vi "Lockin_AIWFM_time.vi"(8 "error in (no error)":errorcluster, 11 "Transport":refnum<class "Transport.lvclass">) -> (0 "error out":errorcluster, 3 "Transport out":refnum<class "Transport.lvclass">)   [LabVIEW 2016, in "Transport.lvclass"]
uses:
  Transport.lvclass
  Control Experiment/Typedefs/Instruments--cluster.ctl
  <userlib>/LevyLab/Krohn Hite 7008/Instrument.KH7008.lvclass
  <userlib>/LevyLab/Lockin-Multichannel/Instrument.Lockin/Instrument.Lockin.lvclass
  <userlib>/LevyLab/Levylab Instruments/Instrument Types/Cryostat/Instrument.Cryostat.lvclass
  <userlib>/LevyLab/Levylab Instruments/Instrument Types/CBridge/Instrument.CBridge.lvclass
  <userlib>/LevyLab/Levylab Instruments/Instrument Types/Optical Delay Line/Instrument.OpticalDelayLine.lvclass
  <userlib>/LevyLab/Levylab Instruments/Instrument Types/Strain/Instrument.Strain.lvclass
  <userlib>/LevyLab/Levylab Instruments/Instrument Types/VNA/Instrument.VNA.lvclass
  <userlib>/LevyLab/Levylab Instruments/Instrument Types/VSource/Instrument.VSource.lvclass
  Transport.lvclass/Transport.ctl
  Control Experiment/Control Experiment.lvclass/Control Experiment.ctl
  <userlib>/LevyLab/XY Utilities/subVIs/Waveform to XY (single).vi
  <userlib>/LevyLab/XY Utilities/subVIs/Get X and Y (single).vi
  <vilib>/Waveform/WDTOps.llb/WDT Append Waveforms DBL.vi
  Control Experiment/Control Experiment.lvclass
  <userlib>/LevyLab/XY Utilities/xy_utilities.lvlib
panel:
  in  "Stop":bool
  in  "Tab Control":enum32{"Control", "Waveform", "Other"}(tab)
  in  "wait (ms)":u32=1000
  in  "Experiment Description":string="cool down\n\n"
  in  "Experiment Folder":string="cooldown"
  out "AI":cluster{dbl[], dbl[]}[](graph)
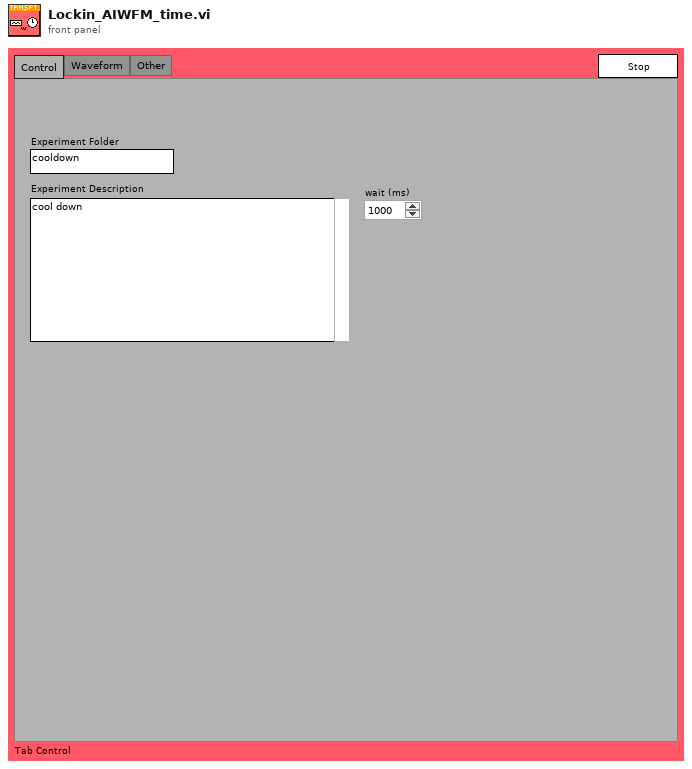
[diagram p1: front panel]
types:
  T1 = enum32{"Invalid", "Standard", "Closed", "Hidden", "Minimized", "Maximized"}
  T2 = enum32{"invalid app kind", "Development System", "Run Time System", "Student Edition", "Embedded LabVIEW", "Evaluation", "Custom"}
  T3 = typedef "Control Experiment.lvclass/Instruments--cluster.ctl" = cluster{"KH7008":refnum<class "Instrument.KH7008.lvclass">[], "Lockin":refnum<class "Instrument.Lockin.lvclass">, "Temperature":refnum<class "Instrument.Cryostat.lvclass">, "Magnet":refnum<class "Instrument.Cryostat.lvclass">, "Rotator":refnum<class "Instrument.Cryostat.lvclass">, "Level":refnum<class "Instrument.Cryostat.lvclass">, "Capacitance Bridge":refnum<class "Instrument.CBridge.lvclass">, "Optical Delay Line":refnum<class "Instrument.OpticalDelayLine.lvclass">, "Strain Cell":refnum<class "Instrument.Strain.lvclass">, "VNA":refnum<class "Instrument.VNA.lvclass">, "Voltage Source":refnum<class "Instrument.VSource.lvclass">}
  T4 = cluster{"Core":cluster{"Current VI Reference":refnum<vi>, "Close Panel on Exit?":bool}, "Transport":refnum<class "Transport.lvclass">, "SweepControl":refnum<class "SweepControl.lvclass">, "Control Experiment":refnum<class "Control Experiment.lvclass">, "Notifier":refnum<notifier>, "Instruments":T3, "path":path, "time":dbl, "temperature":dbl, "magnet field":dbl, "AI XY (new)":cluster{dbl[], dbl[]}[], "AI XY (all)":cluster{dbl[], dbl[]}[], "AI Waveform (s)":waveform(dbl)[], "t0":timestamp}
  T5 = cluster{"Current VI Reference":refnum<vi>, "Close Panel on Exit?":bool}
  T6 = enum32{"Bad", "Idle", "Run top level", "Running"}
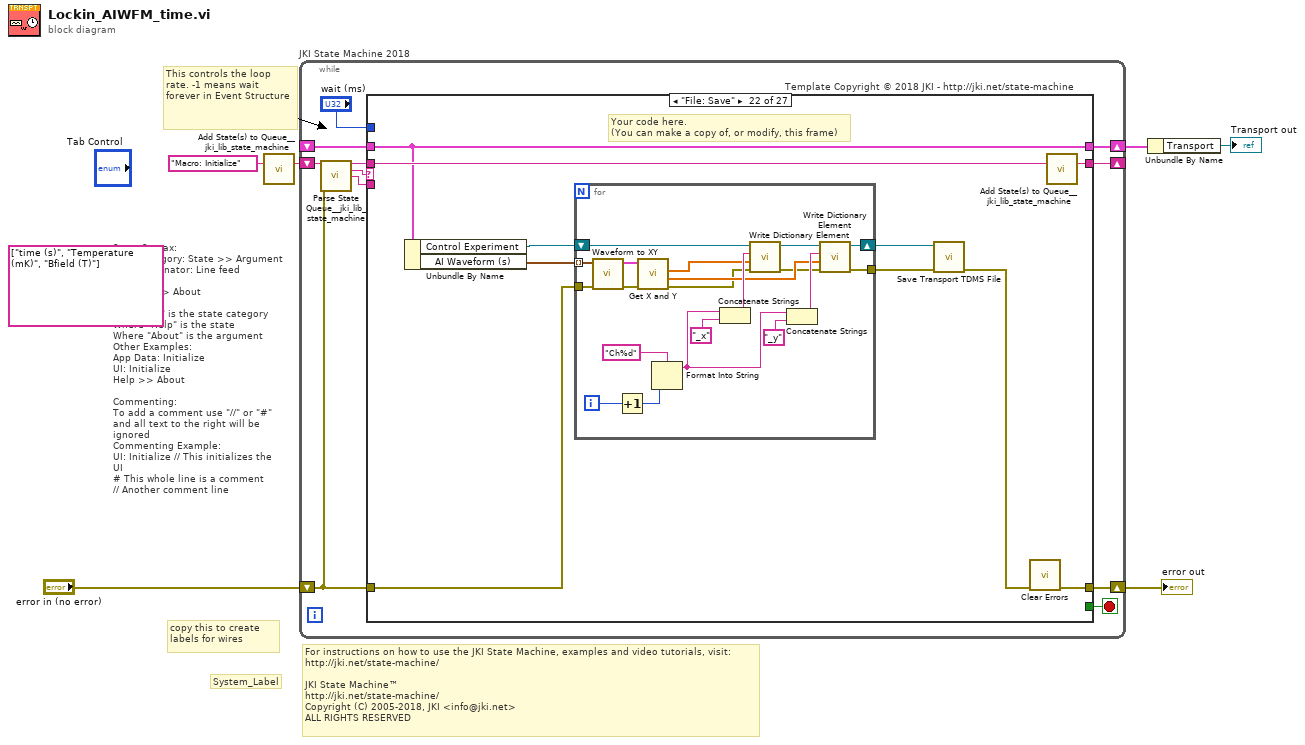
[diagram p0: block diagram]
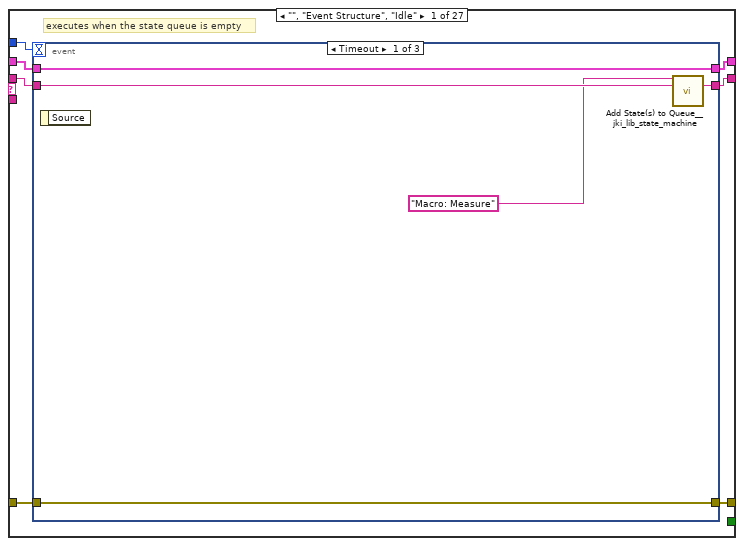
[diagram p2: hidden frame]
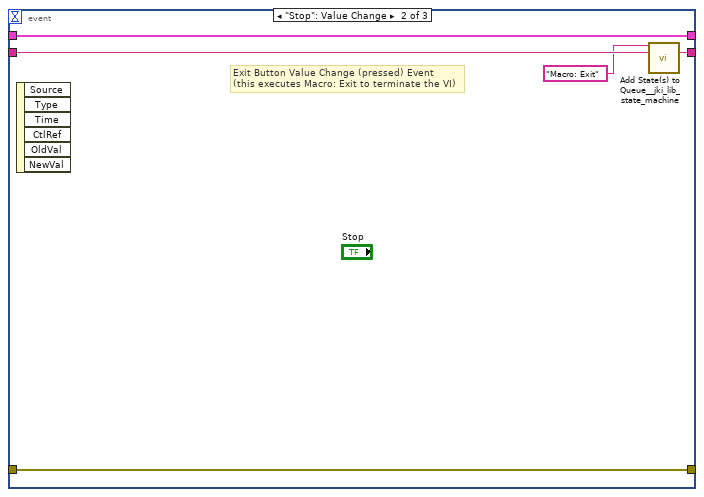
[diagram p3: hidden frame]
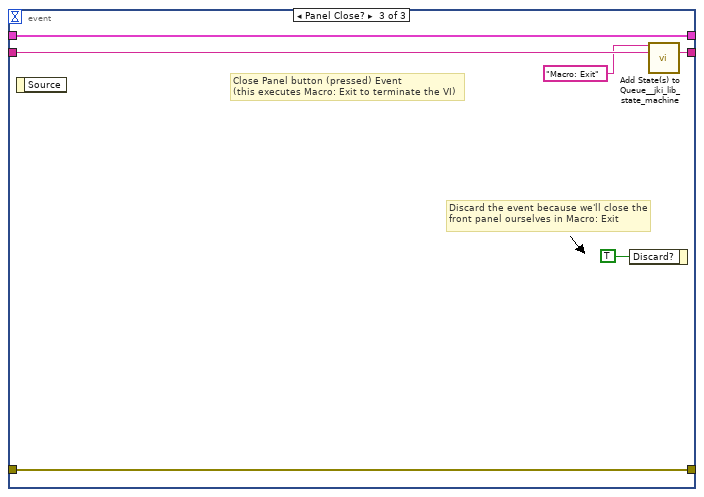
[diagram p4: hidden frame]
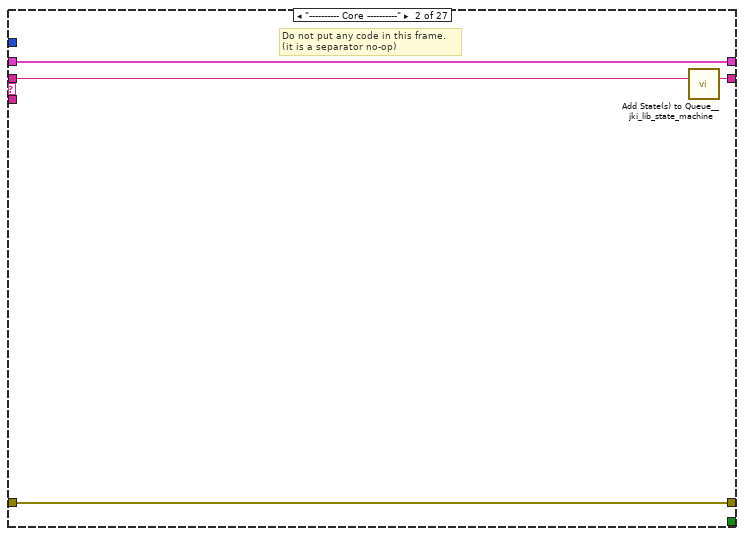
[diagram p5: hidden frame]
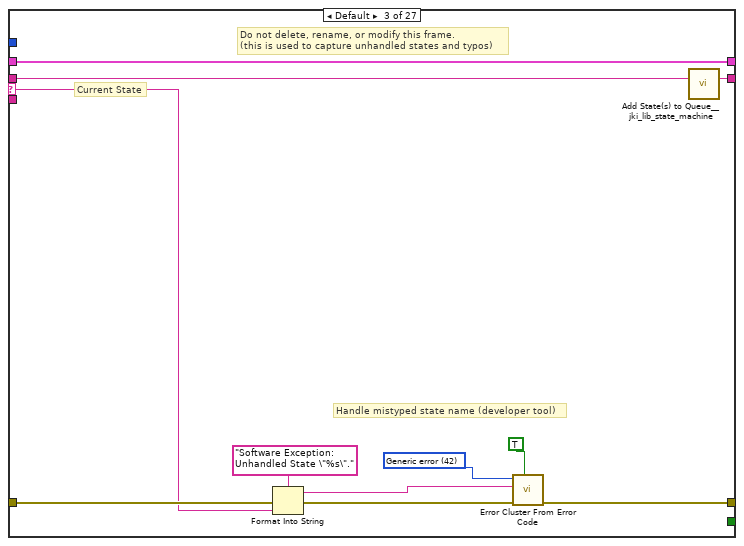
[diagram p6: hidden frame]
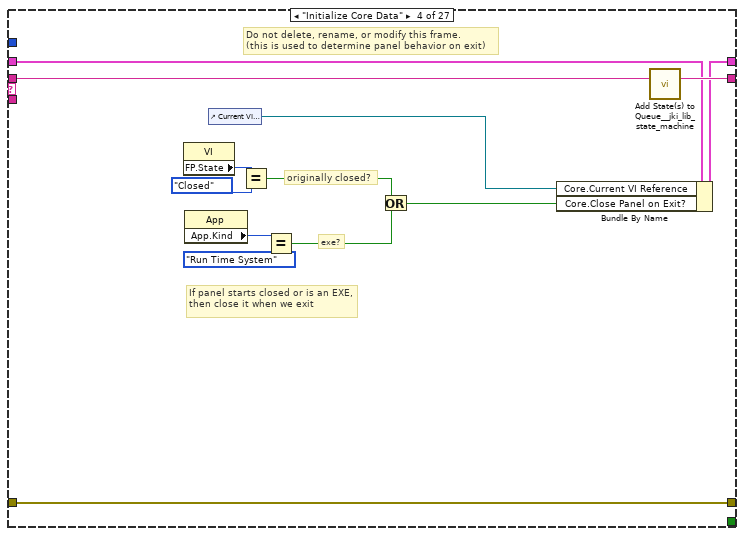
[diagram p7: hidden frame]
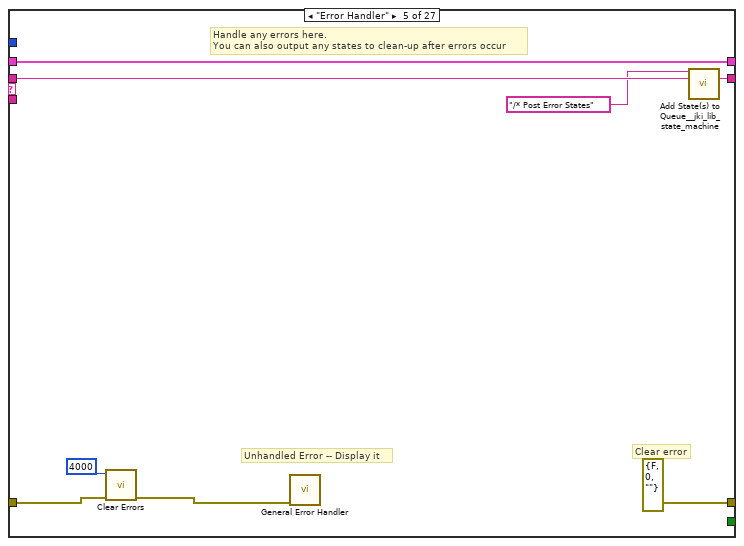
[diagram p8: hidden frame]
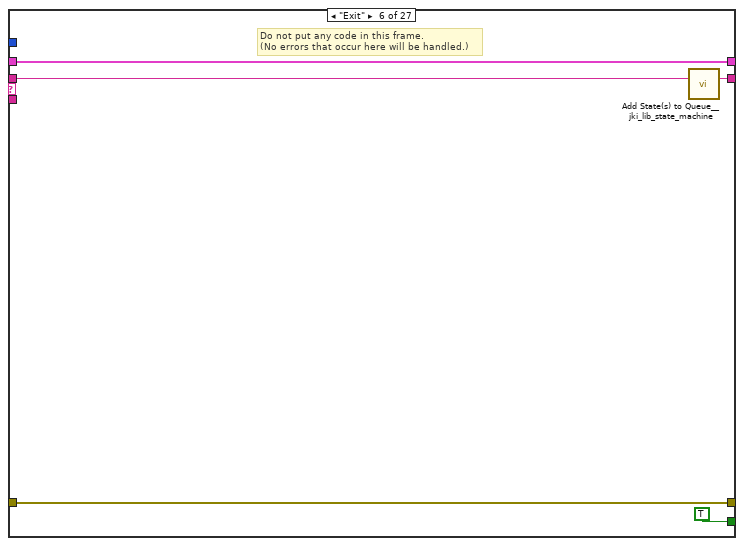
[diagram p9: hidden frame]
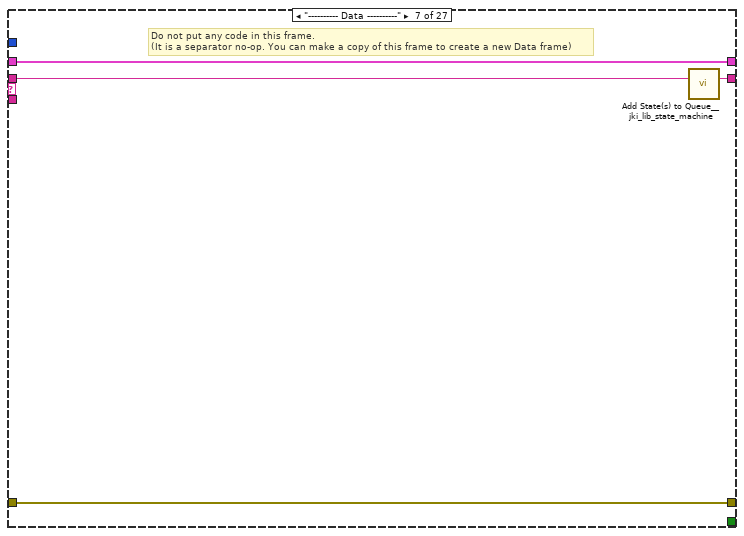
[diagram p10: hidden frame]
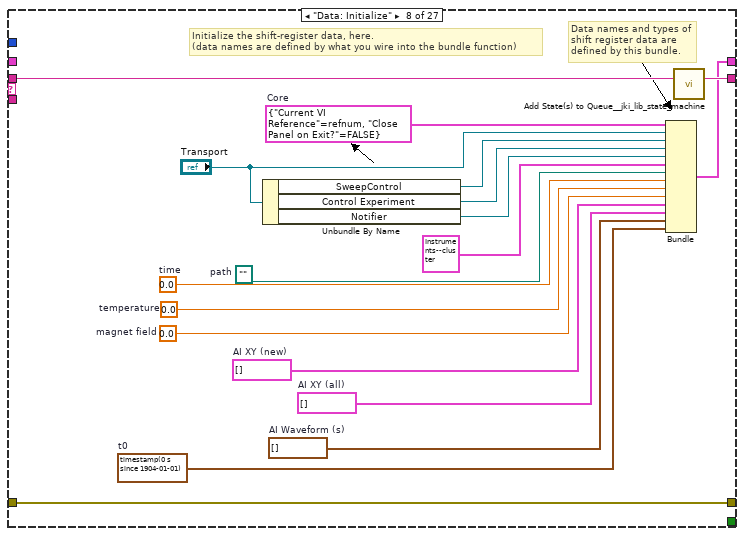
[diagram p11: hidden frame]
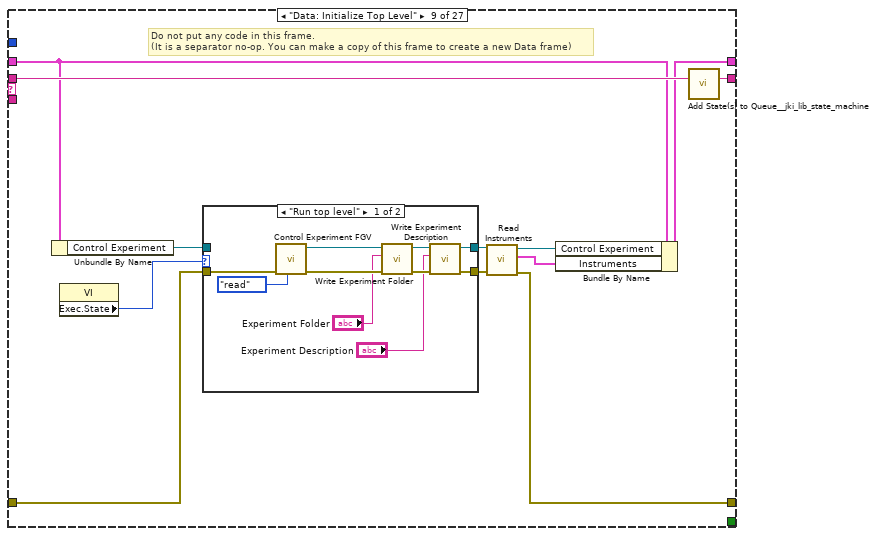
[diagram p12: hidden frame]
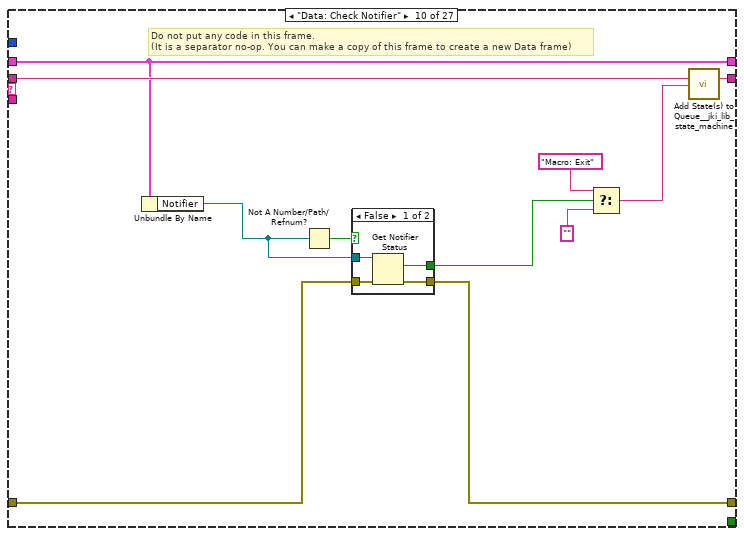
[diagram p14: hidden frame]
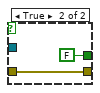
[diagram p15: hidden frame]
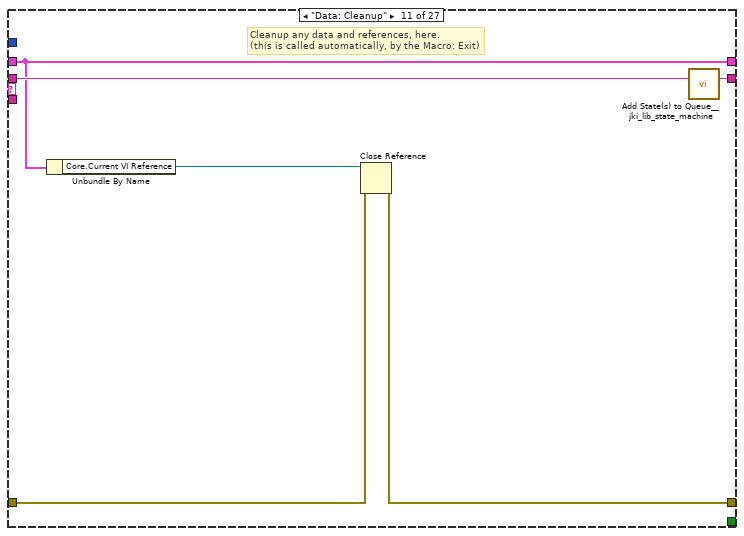
[diagram p16: hidden frame]
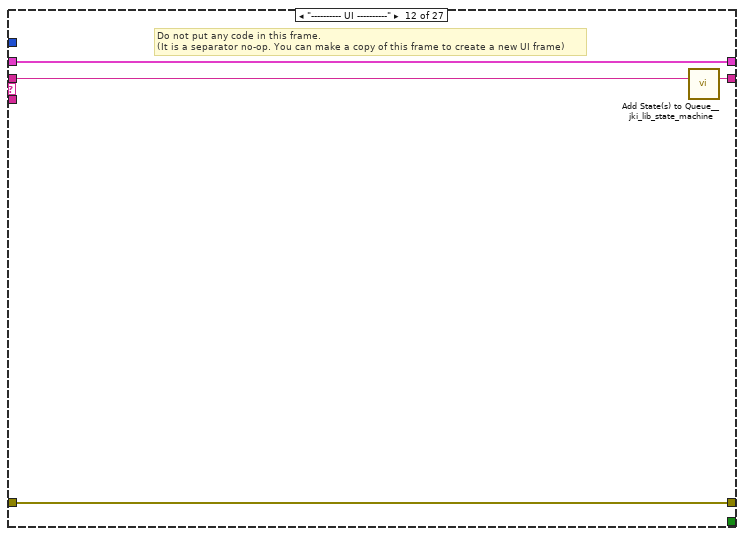
[diagram p17: hidden frame]
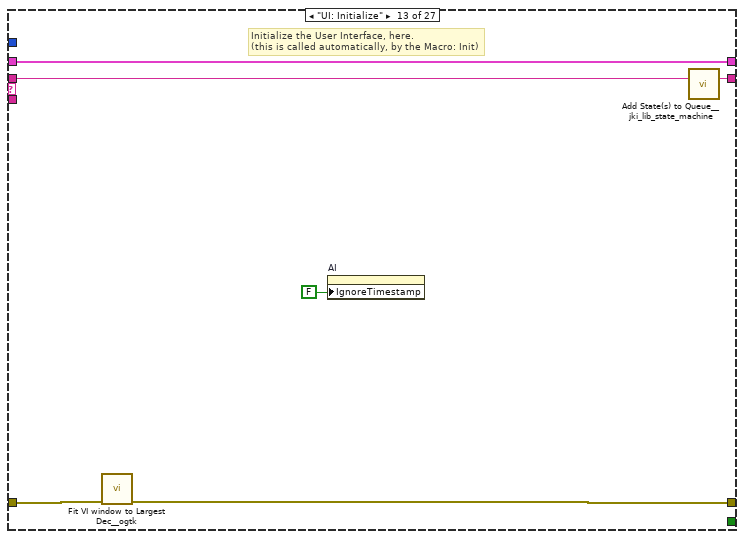
[diagram p18: hidden frame]
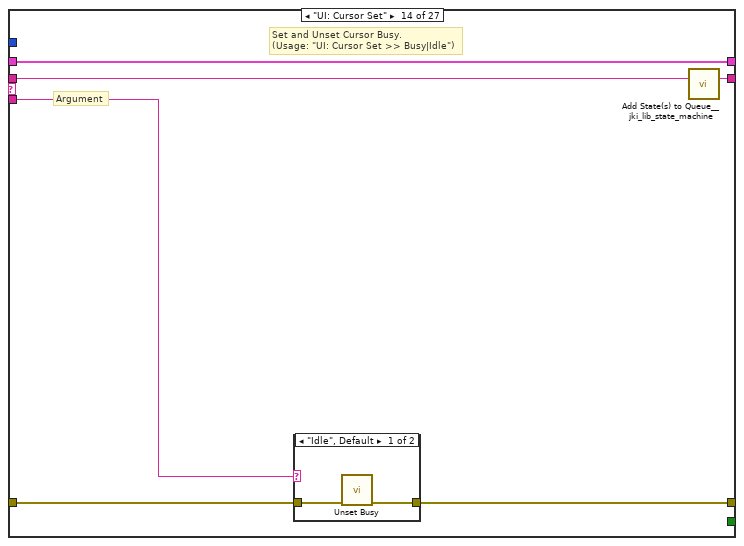
[diagram p19: hidden frame]
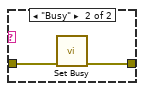
[diagram p20: hidden frame]
diagram:
  (unwired) string[] ["time (s)", "Temperature (mK)", "Bfield (T)"] ("wavenames (.Vx, etc)")
  # "For instructions on how to use the JKI State Machine, examples and video tutorials, visit:\nhttp://jki.net/state-machine/\n\nJKI State Machine™\nhttp://jki.net/state-machine/\nCopyright (C) 2005-2018, JKI <info@jki.net>\nALL RIGHTS RESERVED"
  # "State Syntax:\nStateCategory: State >> Argument\nLine Terminator: Line feed\nExample:\nUI: Help >> About\n\nWhere \"UI\" is the state category\nWhere \"Help\" is the state\nWhere \"About\" is the argument\nOther Examples:\nApp Data: Initialize\nUI: Initialize\nHelp >> About\n\nCommenting:\nTo add a comment use \"//\" or \"#\" and all text to the right will be ignored\nCommenting Example:\nUI: Initialize // This initializes the UI\n# This whole line is a comment\n// Another comment line"
  # "copy this to create labels for wires"
  # "This controls the loop rate. -1 means wait forever in Event Structure"
  # "System_Label"
  n1 = call <vilib>:"Add State(s) to Queue__jki_lib_state_machine.vi"("State(s) in (\"\")"="Macro: Initialize") -> ("States Out"=w6:string)  [unwired: 14 in]
  n2 = while "JKI State Machine 2018" {
    shift-right: [w10] -> w2
    shift-left: _ -> [w9]
    shift-right: [w13] -> w3
    shift-left: "error in (no error)" -> [w8]
    shift-right: [w12] -> _
    shift-left: w6 -> [w14]
    stop <- w11 stop-if-true
    # "Template Copyright © 2018 JKI - http://jki.net/state-machine"
    n3 = call <vilib>:"Parse State Queue__jki_lib_state_machine.vi"("State Queue"=w14, "Error In (no error)"=w8) -> ("Remaining States"=w16:string, "Current State"=w17:string, "Arguments"=w15:string)  [unwired: 11 in]
    n4 = case shown="\"File: Save\"" w17 {
      selector: w17 -> [_ _ w45 _ _ _ _ _ _ _ _ _ _ _ _ _ _ _ _ _ _ _ _ _ _ _ _]
      tunnel: w16 -> [w24 w44 w49 w68 w76 w81 w85 w103 w115 w138 w150 w154 w160 w166 w177 w247 w251 w256 w264 w274 w278 w288 w312 w323 w335 w347 w359]
      tunnel: w15 -> [_ _ _ _ _ _ _ _ _ _ _ _ _ w161 w171 _ _ _ _ _ _ _ _ _ _ _ _]
      tunnel: w9 -> [w22 w41 w47 w61 w73 w79 w82 _ w111 w135 w145 w151 w158 w164 w173 w245 w248 w253 w261 w271 w275 w286 w309 w319 w331 w345 w356]
      tunnel: [w21 w42 w51 w65 errorcluster {"status"=FALSE, "code"=0, "source"=""} ("error out") w78 w83 w100 w105 w133 w146 w152 w156 w162 w174 w244 w249 w254 w262 w272 w276 w285 w310 w313 w324 w340 w350] -> w13
      tunnel: w8 -> [w20 w42 w50 w65 w70 w78 w83 w100 w110 w132 w147 w152 w157 w163 w175 w244 w249 w254 w262 w272 w276 w280 w310 w316 w332 w339 w351]
      tunnel: [w23 w43 w48 w67 w75 w80 w84 w102 w114 w137 w149 w153 w159 w165 w176 w246 w250 w255 w263 w273 w277 w287 w311 w322 w334 w346 w358] -> w12
      tunnel: [_ _ _ _ _ TRUE _ _ _ _ _ _ _ _ _ _ _ _ _ _ _ _ _ _ _ _ _] -> w11
      tunnel: [w19 w41 w47 w66 w73 w79 w82 w101 w112 w135 w145 w151 w158 w164 w173 w245 w248 w253 w261 w271 w275 w286 w309 w320 w330 w344 w357] -> w10
      tunnel: "wait (ms)" -> [w18 _ _ _ _ _ _ _ _ _ _ _ _ _ _ _ _ _ _ _ _ _ _ _ _ _ _]
      frame "", "Event Structure", "Idle" {
        # "executes when the state queue is empty"
        n5 = event shown="[0] Timeout" {
          selector: _ -> [_ _ _]
          dyn-events: _ -> [_ _ _]
          timeout: w18 -> [_ _ _]
          tunnel: w24 -> [w29 w34 w40]
          tunnel: [w28 w33 w39] -> w23
          tunnel: w22 -> [w26 w31 w37]
          tunnel: [w27 w32 w38] -> w21
          tunnel: w20 -> [w27 w32 w38]
          tunnel: [w26 w31 w37] -> w19
          event Timeout {
            n6 = event-data() -> ()  [unwired: 1 in, 1 out]
            n7 = call <vilib>:"Add State(s) to Queue__jki_lib_state_machine.vi"("State(s) in Front (\"\")"="Macro: Measure" ("State(s) in Front (\"\")"), "State(s) in (\"\")"=w29) -> ("States Out"=w28:string)  [unwired: 13 in]
          }
          event "Stop": Value Change {
            # "Exit Button Value Change (pressed) Event\n(this executes Macro: Exit to terminate the VI)"
            n8 = event-data() -> ()  [unwired: 1 in, 6 out]
            n9 = call <vilib>:"Add State(s) to Queue__jki_lib_state_machine.vi"("State(s) in Front (\"\")"="Macro: Exit", "State(s) in (\"\")"=w34) -> ("States Out"=w33:string)  [unwired: 13 in]
          }
          event Panel Close? {
            # "Discard the event because we'll close the front panel ourselves in Macro: Exit"
            # "Close Panel button (pressed) Event\n(this executes Macro: Exit to terminate the VI)"
            n10 = event-data() -> ()  [unwired: 1 in, 1 out]
            n11 = event-data("Discard?"=TRUE) -> ()  [unwired: 1 in, 1 out]
            n12 = call <vilib>:"Add State(s) to Queue__jki_lib_state_machine.vi"("State(s) in Front (\"\")"="Macro: Exit", "State(s) in (\"\")"=w40) -> ("States Out"=w39:string)  [unwired: 13 in]
          }
        }
      }
      frame "---------- Core ----------" {
        # "Do not put any code in this frame.\n(it is a separator no-op)"
        n13 = call <vilib>:"Add State(s) to Queue__jki_lib_state_machine.vi"("State(s) in (\"\")"=w44) -> ("States Out"=w43:string)  [unwired: 14 in]
      }
      frame Default {
        w54 = 42 items=["No error", "Argument error", "Memory is full", "Out of zone", "End of file", "File already open", "Generic file I/O error", "File not found", "File permission error", "Disk is full", "Duplicate path", "Too many files open", "System feature not enabled", "Resource file not found", "Cannot add resource", "Resource not found", "Image not found", "Image memory error", "Pen does not exist", "Config type invalid", "Config token not found", "Config parse error", "Config memory error", "Bad external code format", "Bad external code offset", "External code not present", "Null window", "Destroy window error", "Null menu", "Print aborted", "Bad print record", "Print driver error", "Windows error during printing", "Memory error during printing", "Print dialog error", "Generic print error", "Invalid device refnum", "Device not found", "Device parameter error", "Device unit error", "Cannot open device", "Device call aborted", "Generic error", "Cancelled by user", "Object ID too low", "Object ID too high", "Object not in heap", "Unknown heap", "Unknown object (invalid DefProc)", "Unknown object (DefProc not in table)", "Message out of range", "Invalid (null) method", "Unknown message", "Manager call not supported", "Bad address", "Network operation in progress", "Network operation timed out", "Connection is busy", "Network attribute not supported", "Network error", "Address in use", "System out of memory", "Connection aborted", "Connection refused", "Not connected", "Already connected", "Connection closed", "Initialization error (interapplication manager)", "Bad occurrence", "Wait on unbound occurrence handler", "Occurrence queue overflow", "Datalog type conflict", "Unused", "Unrecognized type (interapplication manager)", "Memory corrupt", "Failed to make temporary DLL", "Old CIN version", "Drag socket not found", "Failed to load drop-object", "Failed to register OLE object", "Failed to release OLE object", "Format specifier type mismatch", "Unknown format specifier", "Too few format specifiers", "Too many format specifiers", "Scan failed", "Newer CIN version", "Error converting to variant", "Runtime menu error", "Password tampered", "Variant attribute not found", "Incompatible variant data type", "Event data is not available", "Event Store is not present", "Occurrence is not found", "Event Queue is not created", "Event info is not available", "Refnum passed is NULL", "Error retrieving Class GUID", "Error retrieving CoClass GUID", "Error retrieving TypeLib GUID.", "Bad built application magic bytes.", "Specific driver is different from the specific driver associated with the Logical Name.", "There is no session opened to the class driver.", "Max Error", "MAX - Error with config objects", "MAX - Error loading configuration", "MAX - Group not supported"]
        # "Current State"
        # "Do not delete, rename, or modify this frame.\n(this is used to capture unhandled states and typos)"
        # "Handle mistyped state name (developer tool)"
        n14 = Format Into String(format string="Software Exception: Unhandled State \"%s\"." ("message"), error in=w50, w45) -> (resulting string=w53:string, error out=w52:errorcluster)  [unwired: 1 in]
        n15 = call <vilib>:"Error Cluster From Error Code.vi"("show call chain? (False)"=TRUE, "error in (no error)"=w52, "error message (\"\")"=w53, "error code (0)"=w54) -> ("error out"=w51:errorcluster)  [unwired: 5 in]
        n16 = call <vilib>:"Add State(s) to Queue__jki_lib_state_machine.vi"("State(s) in (\"\")"=w49) -> ("States Out"=w48:string)  [unwired: 14 in]
      }
      frame "Initialize Core Data" {
        # "Do not delete, rename, or modify this frame.\n(this is used to determine panel behavior on exit)"
        # "originally closed?"
        # "exe?"
        # "If panel starts closed or is an EXE, then close it when we exit"
        n17 = property class="VI"() -> ("FP.State"=w58:T1)  [unwired: 2 in, 2 out]
        n18 = property class="App"() -> ("App.Kind"=w64:T2)  [unwired: 2 in, 2 out]
        n19 = control-ref of="Current VI Reference"() -> (w59:refnum<vi>)
        n20 = Equal?(x=w58, y=T1."Closed" ("Front Panel Window:State")) -> (x = y?=w56:bool)
        n21 = Equal?(x=w64, y=T2."Run Time System" ("Application:Kind")) -> (x = y?=w62:bool)
        n22 = Or(x=w56, y=w62) -> (x .or. y?=w60:bool)
        n23 = Bundle By Name(cluster=w61, "Core.Current VI Reference"=w59, "Core.Close Panel on Exit?"=w60) -> (w66:T4)
        n24 = call <vilib>:"Add State(s) to Queue__jki_lib_state_machine.vi"("State(s) in (\"\")"=w68) -> ("States Out"=w67:string)  [unwired: 14 in]
      }
      frame "Error Handler" {
        # "Unhandled Error -- Display it"
        # "Handle any errors here.\nYou can also output any states to clean-up after errors occur"
        # "Clear error"
        n25 = call <vilib>:"Clear Errors.vi"("error in (no error)"=w70, "specific error code to clear (0: all)"=4000) -> ("error out"=w69:errorcluster)  [unwired: 4 in, 1 out]
        n26 = call <vilib>:"General Error Handler.vi"("error in (no error)"=w69) -> ()  [unwired: 10 in, 5 out]
        n27 = call <vilib>:"Add State(s) to Queue__jki_lib_state_machine.vi"("State(s) in Front (\"\")"="/* Post Error States", "State(s) in (\"\")"=w76) -> ("States Out"=w75:string)  [unwired: 13 in]
      }
      frame "Exit" {
        # "Do not put any code in this frame.\n(No errors that occur here will be handled.)"
        n28 = call <vilib>:"Add State(s) to Queue__jki_lib_state_machine.vi"("State(s) in (\"\")"=w81) -> ("States Out"=w80:string)  [unwired: 14 in]
      }
      frame "---------- Data ----------" {
        # "Do not put any code in this frame.\n(It is a separator no-op. You can make a copy of this frame to create a new Data frame)"
        n29 = call <vilib>:"Add State(s) to Queue__jki_lib_state_machine.vi"("State(s) in (\"\")"=w85) -> ("States Out"=w84:string)  [unwired: 14 in]
      }
      frame "Data: Initialize" {
        w86 = timestamp(0 s since 1904-01-01)  # t0
        w87 = waveform(dbl)[] []  # AI Waveform (s)
        w92 = cluster{dbl[], dbl[]}[] []  # AI XY (new)
        w93 = cluster{dbl[], dbl[]}[] []  # AI XY (all)
        w90 = 0.0  # magnet field
        w89 = 0.0  # temperature
        w88 = 0.0  # time
        w98 = path ""  # path
        w99 = T5 {"Current VI Reference"=refnum, "Close Panel on Exit?"=FALSE}  # Core
        # "Data names and types of shift register data are defined by this bundle."
        # "Initialize the shift-register data, here.\n(data names are defined by what you wire into the bundle function)"
        n30 = Unbundle By Name("Transport") -> ("SweepControl"=w96:refnum<class "SweepControl.lvclass">, "Control Experiment"=w95:refnum<class "Control Experiment.lvclass">, "Notifier"=w94:refnum<notifier>)
        n31 = Bundle("Core"=w99, "Transport"="Transport", "SweepControl"=w96, "Control Experiment"=w95, "Notifier"=w94, "Instruments"=T3 {"KH7008"=[], "Lockin"=refnum, "Temperature"=refnum, "Magnet"=refnum, "Rotator"=refnum, "Level"=refnum, "Capacitance Bridge"=refnum, "Optical Delay Line"=refnum, "Strain Cell"=refnum, "VNA"=refnum, "Voltage Source"=refnum}, "path"=w98, "time"=w88, "temperature"=w89, "magnet field"=w90, "AI XY (new)"=w92, "AI XY (all)"=w93, "AI Waveform (s)"=w87, "t0"=w86) -> (w101:T4)  [unwired: 1 in]
        n32 = call <vilib>:"Add State(s) to Queue__jki_lib_state_machine.vi"("State(s) in (\"\")"=w103) -> ("States Out"=w102:string)  [unwired: 14 in]
      }
      frame "Data: Initialize Top Level" {
        # "Do not put any code in this frame.\n(It is a separator no-op. You can make a copy of this frame to create a new Data frame)"
        n33 = Unbundle By Name(w111) -> ("Control Experiment"=w113:refnum<class "Control Experiment.lvclass">)
        n34 = property class="VI"() -> ("Exec.State"=w104:T6)  [unwired: 2 in, 2 out]
        n35 = case shown="\"Run top level\"" w104 {
          tunnel: w110 -> [w125 w126]
          tunnel: [w120 w126] -> w109
          tunnel: [w119 w127] -> w108
          tunnel: w113 -> [_ w127]
          frame "Run top level" {
            n36 = call "Control Experiment FGV.vi"("Function"=enum16{"read", "write"}."read", "error in (no error)"=w125) -> ("error out"=w123:errorcluster, "Control Experiment.lvclass out"=w124:refnum<class "Control Experiment.lvclass">)  [unwired: 8 in]
            n37 = call "Write Experiment Folder.vi"("error in (no error)"=w123, "Experiment Folder"="Experiment Folder", "Control Experiment in"=w124) -> ("error out"=w121:errorcluster, "Control Experiment out"=w122:refnum<class "Control Experiment.lvclass">)  [unwired: 7 in]
            n38 = call "Write Experiment Description.vi"("error in (no error)"=w121, "Experiment Description"="Experiment Description", "Control Experiment in"=w122) -> ("error out"=w120:errorcluster, "Control Experiment out"=w119:refnum<class "Control Experiment.lvclass">)  [unwired: 7 in]
          }
          frame "Running", Default {
          }
        }
        n39 = call "Read Instruments.vi"("error in (no error)"=w109, "Control Experiment in"=w108) -> ("error out"=w105:errorcluster, "Instruments"=w106:T3, "Control Experiment out"=w107:refnum<class "Control Experiment.lvclass">)  [unwired: 7 in]
        n40 = Bundle By Name(cluster=w111, "Control Experiment"=w107, "Instruments"=w106) -> (w112:T4)
        n41 = call <vilib>:"Add State(s) to Queue__jki_lib_state_machine.vi"("State(s) in (\"\")"=w115) -> ("States Out"=w114:string)  [unwired: 14 in]
      }
      frame "Data: Check Notifier" {
        # "Do not put any code in this frame.\n(It is a separator no-op. You can make a copy of this frame to create a new Data frame)"
        n42 = Unbundle By Name(w135) -> ("Notifier"=w134:refnum<notifier>)
        n43 = Not A Number/Path/Refnum?(number/path/refnum=w134) -> (NaN/Path/Refnum?=w136:bool)
        n44 = case shown="False" w136 {
          tunnel: [w142 FALSE] -> w131
          tunnel: [w141 w143] -> w133
          tunnel: w134 -> [w140 _]
          tunnel: w132 -> [w139 w143]
          frame False {
            n45 = Get Notifier Status(notifier=w140, error in (no error)=w139) -> (current notification=w142:bool, error out=w141:errorcluster)  [unwired: 3 out]
          }
          frame True {
          }
        }
        n46 = Select(t="Macro: Exit", s=w131, f="") -> (s? t:f=w128:string)
        n47 = call <vilib>:"Add State(s) to Queue__jki_lib_state_machine.vi"("State(s) in (\"\")"=w138, "State(s) at Back (\"\")"=w128) -> ("States Out"=w137:string)  [unwired: 13 in]
      }
      frame "Data: Cleanup" {
        # "Cleanup any data and references, here.\n(this is called automatically, by the Macro: Exit)"
        n48 = Unbundle By Name(w145) -> ("Core.Current VI Reference"=w148:refnum<vi>)
        n49 = Close Reference(reference=w148, error in (no error)=w147) -> (error out=w146:errorcluster)
        n50 = call <vilib>:"Add State(s) to Queue__jki_lib_state_machine.vi"("State(s) in (\"\")"=w150) -> ("States Out"=w149:string)  [unwired: 14 in]
      }
      frame "---------- UI ----------" {
        # "Do not put any code in this frame.\n(It is a separator no-op. You can make a copy of this frame to create a new UI frame)"
        n51 = call <vilib>:"Add State(s) to Queue__jki_lib_state_machine.vi"("State(s) in (\"\")"=w154) -> ("States Out"=w153:string)  [unwired: 14 in]
      }
      frame "UI: Initialize" {
        # "Initialize the User Interface, here.\n(this is called automatically, by the Macro: Init)"
        n52 = call <userlib>:"Fit VI window to Largest Dec__ogtk.vi"("error in (no error)"=w157) -> ("error out"=w156:errorcluster)  [unwired: 5 in, 1 out]
        n53 = property on="AI" class="XYGraph (strict)"("IgnoreTimestamp"=FALSE ("Ignore Timestamp")) -> ()  [unwired: 2 in, 2 out]
        n54 = call <vilib>:"Add State(s) to Queue__jki_lib_state_machine.vi"("State(s) in (\"\")"=w160) -> ("States Out"=w159:string)  [unwired: 14 in]
      }
      frame "UI: Cursor Set" {
        # "Argument"
        # "Set and Unset Cursor Busy.\n(Usage: \"UI: Cursor Set >> Busy|Idle\")"
        n55 = case shown="\"Idle\", Default" w161 {
          tunnel: w163 -> [w168 w170]
          tunnel: [w167 w169] -> w162
          frame "Idle", Default {
            n56 = call <vilib>:"Unset Busy.vi"("error in (no error)"=w168) -> ("error out"=w167:errorcluster)  [unwired: 10 in]
          }
          frame "Busy" {
            n57 = call <vilib>:"Set Busy.vi"("error in (no error)"=w170) -> ("error out"=w169:errorcluster)  [unwired: 9 in, 1 out]
          }
        }
        n58 = call <vilib>:"Add State(s) to Queue__jki_lib_state_machine.vi"("State(s) in (\"\")"=w166) -> ("States Out"=w165:string)  [unwired: 14 in]
      }
      frame "UI: Front Panel State" {
        # "Argument"
        # "Set Front Panel Open or Closed\n(Usage: \"UI: Front Panel State >> Open|Close\")"
        n59 = Unbundle By Name(w173) -> ("Core.Current VI Reference"=w172:refnum<vi>)
        n60 = case shown="\"Minimize\", \"Minimized\"" w171 {
          tunnel: w175 -> [w183 w198 w209 w222 w235]
          tunnel: [w185 w199 w211 w224 w237] -> w174
          tunnel: w172 -> [w184 w196 w210 w223 w236]
          frame "Open", "Standard", Default {
            w178 = T1."Standard" ("State")
            n61 = property class="VI"(reference=w184, error in=w183) -> (reference out=w181:refnum<vi>, error out=w182:errorcluster, "FP.State"=w180:T1)
            n62 = Not Equal?(x=w180, y=w178) -> (x != y?=w179:bool)
            n63 = case shown="True" w179 {
              tunnel: [w189 w191] -> w185
              tunnel: w182 -> [w188 w191]
              tunnel: w181 -> [w187 _]
              tunnel: w178 -> [w186 _]
              frame True {
                n64 = invoke class="VI" method="FP.Open"(reference=w187, error in=w188, "Activate"=TRUE, "State"=w186) -> (error out=w189:errorcluster)  [unwired: 1 in, 4 out]
              }
              frame False {
              }
            }
          }
          frame "Close", "Closed" {
            n65 = property class="VI"(reference=w196, error in=w198) -> (reference out=w195:refnum<vi>, error out=w197:errorcluster, "FP.State"=w193:T1)
            n66 = Not Equal?(x=w193, y=T1."Closed" ("Front Panel Window:State")) -> (x != y?=w192:bool)
            n67 = case shown="True" w192 {
              tunnel: [w200 w203] -> w199
              tunnel: w197 -> [w200 w202]
              tunnel: w195 -> [_ w201]
              frame False {
              }
              frame True {
                n68 = invoke class="VI" method="FP.Close"(reference=w201, error in=w202) -> (error out=w203:errorcluster)  [unwired: 1 in, 2 out]
              }
            }
          }
          frame "Hidden", "Hide" {
            w204 = T1."Hidden" ("State")
            n69 = property class="VI"(reference=w210, error in=w209) -> (reference out=w207:refnum<vi>, error out=w208:errorcluster, "FP.State"=w206:T1)
            n70 = Not Equal?(x=w206, y=w204) -> (x != y?=w205:bool)
            n71 = case shown="True" w205 {
              tunnel: [w215 w216] -> w211
              tunnel: w208 -> [w214 w216]
              tunnel: w207 -> [w213 _]
              tunnel: w204 -> [w212 _]
              frame True {
                n72 = invoke class="VI" method="FP.Open"(reference=w213, error in=w214, "State"=w212) -> (error out=w215:errorcluster)  [unwired: 2 in, 4 out]
              }
              frame False {
              }
            }
          }
          frame "Minimize", "Minimized" {
            w217 = T1."Minimized" ("State")
            n73 = property class="VI"(reference=w223, error in=w222) -> (reference out=w220:refnum<vi>, error out=w221:errorcluster, "FP.State"=w219:T1)
            n74 = Not Equal?(x=w219, y=w217) -> (x != y?=w218:bool)
            n75 = case shown="True" w218 {
              tunnel: [w228 w229] -> w224
              tunnel: w221 -> [w227 w229]
              tunnel: w220 -> [w226 _]
              tunnel: w217 -> [w225 _]
              frame True {
                n76 = invoke class="VI" method="FP.Open"(reference=w226, error in=w227, "State"=w225) -> (error out=w228:errorcluster)  [unwired: 2 in, 4 out]
              }
              frame False {
              }
            }
          }
          frame "Maximize", "Maximized" {
            w230 = T1."Maximized" ("State")
            n77 = property class="VI"(reference=w236, error in=w235) -> (reference out=w233:refnum<vi>, error out=w234:errorcluster, "FP.State"=w232:T1)
            n78 = Not Equal?(x=w232, y=w230) -> (x != y?=w231:bool)
            n79 = case shown="True" w231 {
              tunnel: [w241 w242] -> w237
              tunnel: w234 -> [w240 w242]
              tunnel: w233 -> [w239 _]
              tunnel: w230 -> [w238 _]
              frame True {
                n80 = invoke class="VI" method="FP.Open"(reference=w239, error in=w240, "State"=w238) -> (error out=w241:errorcluster)  [unwired: 2 in, 4 out]
              }
              frame False {
              }
            }
          }
        }
        n81 = call <vilib>:"Add State(s) to Queue__jki_lib_state_machine.vi"("State(s) in (\"\")"=w177) -> ("States Out"=w176:string)  [unwired: 14 in]
      }
      frame "UI: Update Graphs" {
        # "Do not put any code in this frame.\n(It is a separator no-op. You can make a copy of this frame to create a new UI frame)"
        n82 = Unbundle By Name(w245) -> ("AI XY (all)"=→"AI":cluster{dbl[], dbl[]}[])
        n83 = call <vilib>:"Add State(s) to Queue__jki_lib_state_machine.vi"("State(s) in (\"\")"=w247) -> ("States Out"=w246:string)  [unwired: 14 in]
      }
      frame "---------- Macro ----------" {
        # "Do not put any code in this frame.\n(It is a separator no-op. You can make a copy of this frame to create a new Macro frame)"
        n84 = call <vilib>:"Add State(s) to Queue__jki_lib_state_machine.vi"("State(s) in (\"\")"=w251) -> ("States Out"=w250:string)  [unwired: 14 in]
      }
      frame "Macro: Initialize" {
        w252 = "Data: Initialize\nInitialize Core Data\nUI: Initialize\nUI: Front Panel State >> Open\nData: Initialize Top Level"  # Data: Initialize Initialize Core Data UI: Initialize UI: Front Panel State >> Open Data: Initialize Top Level
        # "Initialization Macro\n(This is called once, when the VI starts)"
        n85 = call <vilib>:"Add State(s) to Queue__jki_lib_state_machine.vi"("State(s) in Front (\"\")"=w252, "State(s) in (\"\")"=w256) -> ("States Out"=w255:string)  [unwired: 13 in]
      }
      frame "Macro: Measure" {
        # "Initialization Macro\n(This is called once, when the VI starts)"
        n86 = call <vilib>:"Add State(s) to Queue__jki_lib_state_machine.vi"("State(s) in Front (\"\")"="Measure: Time\nMeasure: Temperature\nMeasure: Magnet\nMeasure: Lockin\nUI: Update Graphs", "State(s) in (\"\")"="File: Save", "State(s) at Back (\"\")"="Data: Check Notifier") -> ("States Out"=w259:string)  [unwired: 12 in]
        n87 = call <vilib>:"Add State(s) to Queue__jki_lib_state_machine.vi"("State(s) in Front (\"\")"=w259, "State(s) in (\"\")"=w264) -> ("States Out"=w263:string)  [unwired: 13 in]
      }
      frame "Macro: Exit" {
        # "Exit Macro\n(This is called once, when the VI exits)"
        n88 = Unbundle By Name(w271) -> ("Core.Close Panel on Exit?"=w270:bool)
        n89 = Select(t="UI: Front Panel State >> Close", s=w270, f="") -> (s? t:f=w267:string)
        n90 = call <vilib>:"Add State(s) to Queue__jki_lib_state_machine.vi"("State(s) in (\"\")"=w267, "State(s) at Back (\"\")"="Data: Cleanup\nExit") -> ("States Out"=w265:string)  [unwired: 13 in]
        n91 = call <vilib>:"Add State(s) to Queue__jki_lib_state_machine.vi"("State(s) in Front (\"\")"=w265, "State(s) in (\"\")"=w274) -> ("States Out"=w273:string)  [unwired: 13 in]
      }
      frame "---------- File ----------" {
        # "Template Separator\n(You can make a copy of, or modify, this frame)"
        n92 = call <vilib>:"Add State(s) to Queue__jki_lib_state_machine.vi"("State(s) in (\"\")"=w278) -> ("States Out"=w277:string)  [unwired: 14 in]
      }
      frame "File: Save" {
        # "Your code here.\n(You can make a copy of, or modify, this frame)"
        n93 = Unbundle By Name(w286) -> ("Control Experiment"=w282:refnum<class "Control Experiment.lvclass">, "AI Waveform (s)"=w283:waveform(dbl)[])
        n94 = for {
          tunnel: w283 -> [w306] mode=indexing
          tunnel: w280 -> [w305]
          shift-right: [w290] -> w281
          shift-left: w282 -> [w301]
          tunnel: [w289] -> w279
          i -> [w298]
          n95 = call-poly <userlib>:"Waveform to XY.vi"("error in (no error)"=w305, "Waveform in"=w306) -> ("error out"=w307:errorcluster, "XY-data out"=w308:cluster{"X-array":dbl[], "Y-array":dbl[]})  [unwired: 8 in]
          n96 = Increment(x=w298) -> (x+1=w300:i32)
          n97 = call-poly <userlib>:"Get X and Y.vi"("error in (no error)"=w307, "XY-data"=w308) -> ("error out"=w292:errorcluster, "Y-array"=w293:dbl[], "X-array"=w294:dbl[])  [unwired: 6 in, 1 out]
          n98 = Format Into String(format string="Ch%d" ("wavenames"), w300) -> (resulting string=w297:string)  [unwired: 2 in, 1 out]
          n99 = Concatenate Strings(w297, "_x" ("string")) -> (w303:string)
          n100 = call "Write Dictionary Element.vi"("error in (no error)"=w292, "value"=w294, "key"=w303, "Control Experiment in"=w301) -> ("error out"=w291:errorcluster, "Control Experiment out"=w302:refnum<class "Control Experiment.lvclass">)  [unwired: 6 in]
          n101 = Concatenate Strings(w297, "_y" ("string")) -> (w304:string)
          n102 = call "Write Dictionary Element.vi"("error in (no error)"=w291, "value"=w293, "key"=w304, "Control Experiment in"=w302) -> ("error out"=w289:errorcluster, "Control Experiment out"=w290:refnum<class "Control Experiment.lvclass">)  [unwired: 6 in]
        }
        n103 = call "Save Transport TDMS File.vi"("error in (no error)"=w279, "Control Experiment in"=w281) -> ("error out"=w284:errorcluster)  [unwired: 8 in, 1 out]
        n104 = call <vilib>:"Clear Errors.vi"("error in (no error)"=w284) -> ("error out"=w285:errorcluster)  [unwired: 5 in, 1 out]
        n105 = call <vilib>:"Add State(s) to Queue__jki_lib_state_machine.vi"("State(s) in (\"\")"=w288) -> ("States Out"=w287:string)  [unwired: 14 in]
      }
      frame "---------- Measure ----------" {
        # "Do not put any code in this frame.\n(It is a separator no-op. You can make a copy of this frame to create a new Macro frame)"
        n106 = call <vilib>:"Add State(s) to Queue__jki_lib_state_machine.vi"("State(s) in (\"\")"=w312) -> ("States Out"=w311:string)  [unwired: 14 in]
      }
      frame "Measure: Time" {
        # "Do not put any code in this frame.\n(It is a separator no-op. You can make a copy of this frame to create a new Macro frame)"
        n107 = Unbundle By Name(w319) -> ("Control Experiment"=w318:refnum<class "Control Experiment.lvclass">)
        n108 = Get Date/Time In Seconds() -> (seconds since 1Jan1904=w321:timestamp)
        n109 = To Double Precision Float(number=w321) -> (double precision float=w314:dbl)
        n110 = call "Append Dictionary Element.vi"("error in (no error)"=w316, "value"=w314, "key"="Time", "Control Experiment in"=w318) -> ("error out"=w313:errorcluster, "Control Experiment out"=w317:refnum<class "Control Experiment.lvclass">)  [unwired: 6 in]
        n111 = Bundle By Name(cluster=w319, "Control Experiment"=w317) -> (w320:T4)
        n112 = call <vilib>:"Add State(s) to Queue__jki_lib_state_machine.vi"("State(s) in (\"\")"=w323) -> ("States Out"=w322:string)  [unwired: 14 in]
      }
      frame "Measure: Temperature" {
        # "Do not put any code in this frame.\n(It is a separator no-op. You can make a copy of this frame to create a new Macro frame)"
        n113 = Unbundle By Name(w331) -> ("Control Experiment"=w326:refnum<class "Control Experiment.lvclass">, "Instruments.Temperature"=w333:refnum<class "Instrument.Cryostat.lvclass">)
        n114 = call-dynamic "Get Temperature.vi"("error in (no error)"=w332, "Instrument.Cryostat in"=w333) -> ("error out"=w327:errorcluster, "Temperature (K)"=w328:dbl)  [unwired: 5 in, 3 out]
        n115 = call "Append Dictionary Element.vi"("error in (no error)"=w327, "value"=w328, "key"="Temperature", "Control Experiment in"=w326) -> ("error out"=w324:errorcluster, "Control Experiment out"=w325:refnum<class "Control Experiment.lvclass">)  [unwired: 6 in]
        n116 = Bundle By Name(cluster=w331, "Control Experiment"=w325) -> (w330:T4)
        n117 = call <vilib>:"Add State(s) to Queue__jki_lib_state_machine.vi"("State(s) in (\"\")"=w335) -> ("States Out"=w334:string)  [unwired: 14 in]
      }
      frame "Measure: Magnet" {
        # "Do not put any code in this frame.\n(It is a separator no-op. You can make a copy of this frame to create a new Macro frame)"
        n118 = Unbundle By Name(w345) -> ("Control Experiment"=w342:refnum<class "Control Experiment.lvclass">, "Instruments.Temperature"=w337:refnum<class "Instrument.Cryostat.lvclass">)
        n119 = call-dynamic "Get Magnet Field.vi"("error in (no error)"=w339, "Instrument.Cryostat in"=w337) -> ("error out"=w338:errorcluster, "B Field (T)"=w336:dbl)  [unwired: 5 in, 3 out]
        n120 = call "Append Dictionary Element.vi"("error in (no error)"=w338, "value"=w336, "key"="Magnet", "Control Experiment in"=w342) -> ("error out"=w340:errorcluster, "Control Experiment out"=w341:refnum<class "Control Experiment.lvclass">)  [unwired: 6 in]
        n121 = Bundle By Name(cluster=w345, "Control Experiment"=w341) -> (w344:T4)
        n122 = call <vilib>:"Add State(s) to Queue__jki_lib_state_machine.vi"("State(s) in (\"\")"=w347) -> ("States Out"=w346:string)  [unwired: 14 in]
      }
      frame "Measure: Lockin" {
        # "Do not put any code in this frame.\n(It is a separator no-op. You can make a copy of this frame to create a new Macro frame)"
        n123 = Unbundle By Name(w356) -> ("t0"=w353:timestamp, "AI Waveform (s)"=w349:waveform(dbl)[], "Instruments.Lockin"=w352:refnum<class "Instrument.Lockin.lvclass">)
        n124 = Array Size(array=w349) -> (size(s)=w348:i32)
        n125 = case shown="Default" w348 {
          tunnel: w349 -> [w363 w382]
          tunnel: [w363 w381] -> w355
          tunnel: [w365 w380] -> w350
          tunnel: w351 -> [w366 w379]
          tunnel: [w361 w375] -> w354
          tunnel: w352 -> [w367 w374]
          tunnel: w353 -> [_ w372]
          frame 0 {
            n126 = for {
              N: 3 -> [_]
              tunnel: w367 -> [w371]
              tunnel: [w368] -> w360
              shift-right: [w369] -> w365
              shift-left: w366 -> [w370]
              n127 = call <userlib>:"waitForNewWaveforms.vi"("error in (no error)"=w370, "Instrument.Lockin in"=w371) -> ("error out"=w369:errorcluster, "Newest AI Waveform"=w368:waveform(dbl)[])  [unwired: 7 in, 1 out]
            }
            n128 = Index Array(array=w360) -> (element=w364:waveform(dbl))  [unwired: 1 in]
            n129 = Unbundle By Name(w364) -> ("t0"=w361:timestamp)
          }
          frame Default {
            n130 = call <userlib>:"getAI.vi"("error in (no error)"=w379, "Instrument.Lockin in"=w374) -> ("error out"=w378:errorcluster, "AI Waveform"=w373:waveform(dbl)[])  [unwired: 7 in, 1 out]
            n131 = Index Array(array=w373) -> (element=w377:waveform(dbl))  [unwired: 1 in]
            n132 = Unbundle By Name(w377) -> ("t0"=w375:timestamp)
            n133 = Equal?(x=w375, y=w372) -> (x = y?=w376:bool)
            n134 = case shown="False" w376 {
              tunnel: w382 -> [w384 w401]
              tunnel: [w387 w401] -> w381
              tunnel: [w386 w402] -> w380
              tunnel: w378 -> [w385 w402]
              tunnel: w373 -> [w388 _]
              frame False {
                n135 = Array Size(array=w384) -> (size(s)=w383:i32)
                n136 = case shown="Default" w383 {
                  tunnel: w388 -> [w390 w395]
                  tunnel: [w390 w394] -> w387
                  tunnel: [w389 w393] -> w386
                  tunnel: w385 -> [w389 w392]
                  tunnel: w384 -> [_ w391]
                  frame 0 {
                  }
                  frame Default {
                    n137 = for {
                      tunnel: w391 -> [w396] mode=indexing
                      tunnel: w395 -> [w400] mode=indexing
                      tunnel: [w399] -> w394 mode=indexing
                      tunnel: [w398] -> w393
                      tunnel: w392 -> [w397]
                      n138 = call-poly <vilib>:"Append Waveforms.vi"("error in (no error)"=w397, "waveform B"=w400, "waveform A"=w396) -> ("error out"=w398:errorcluster, "waveform out"=w399:waveform(dbl))  [unwired: 7 in]
                    }
                  }
                }
              }
              frame True {
              }
            }
          }
        }
        n139 = Bundle By Name(cluster=w356, "t0"=w354, "AI Waveform (s)"=w355) -> (w357:T4)
        n140 = call <vilib>:"Add State(s) to Queue__jki_lib_state_machine.vi"("State(s) in (\"\")"=w359) -> ("States Out"=w358:string)  [unwired: 14 in]
      }
    }
  }
  "error out" <- w3
  n141 = Unbundle By Name(w2) -> ("Transport"=→"Transport out":refnum<class "Transport.lvclass">)
